vi "System Exec Open Command Prompt.vi"   [LabVIEW 2011]
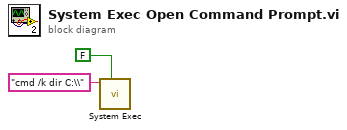
[diagram p0: block diagram]
diagram:
  n1 = call <vilib>:"System Exec.vi"("wait until completion? (T)"=FALSE, "command line"="cmd /k dir C:\\") -> ()  [unwired: 6 in, 4 out]
